vi "Autonomous Output Data.vi"() -> ()   [LabVIEW 2014]
uses:
  Subsystems VIs/Robot Commands.ctl
panel:
  out "Robot System Functions":T1
  # "Field Centric"
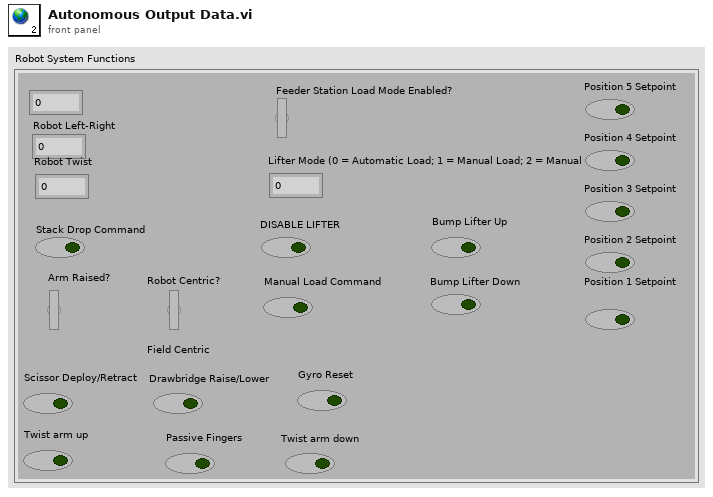
[diagram p1: front panel]
types:
  T1 = typedef "Robot Commands.ctl" = cluster{"Robot Forward-Reverse":dbl, "Robot Left-Right":dbl, "Robot Twist":dbl, "Feeder Station Load Mode Enabled?":bool, "Lifter Mode (0 = Automatic Load; 1 = Manual Load; 2 = Manual Override)":dbl, "Stack Drop Command":bool, "Arm Raised?":bool, "DISABLE LIFTER":bool, "Position 1 Setpoint":bool, "Position 2 Setpoint":bool, "Position 3 Setpoint":bool, "Position 4 Setpoint":bool, "Position 5 Setpoint":bool, "Bump Lifter Down":bool, "Bump Lifter Up":bool, "Manual Load Command":bool, "Robot Centric?":bool, "Scissor Deploy/Retract":bool, "Passive Fingers":bool, "Drawbridge Raise/Lower":bool, "Twist arm up":bool, "Gyro Reset":bool, "Twist arm down":bool}
diagram:
